vi "setVolumeCount.vi"(8 "error in (no error)":errorcluster, 10 "VolumeCount":u32, 11 "VGS_Project in":refnum<class "VGS_Project.lvclass">) -> (0 "error out":errorcluster, 3 "VGS_Project out":refnum<class "VGS_Project.lvclass">)   [LabVIEW 2022 SP3, in "LV_VGS.lvlib" / "VGS_Project.lvclass"]
uses:
  VGS_Project.lvclass
  VGS_Project.lvclass/VGS_Project.ctl
  C:/Users/Andrey/Desktop/hajo/LV_VGS/vgs_project.dll
  vgs_project.dll
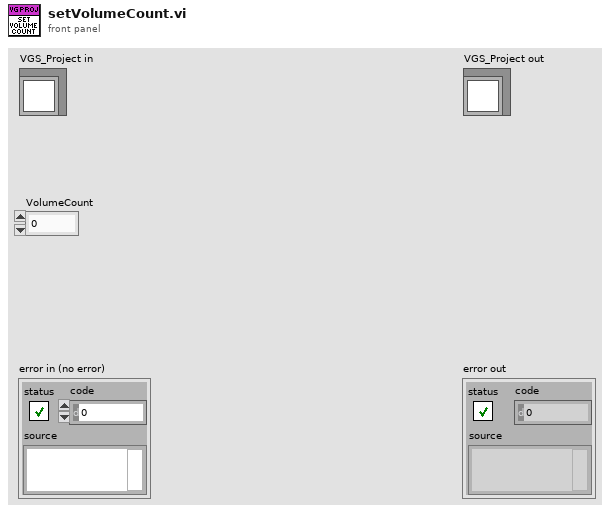
[diagram p1: front panel]
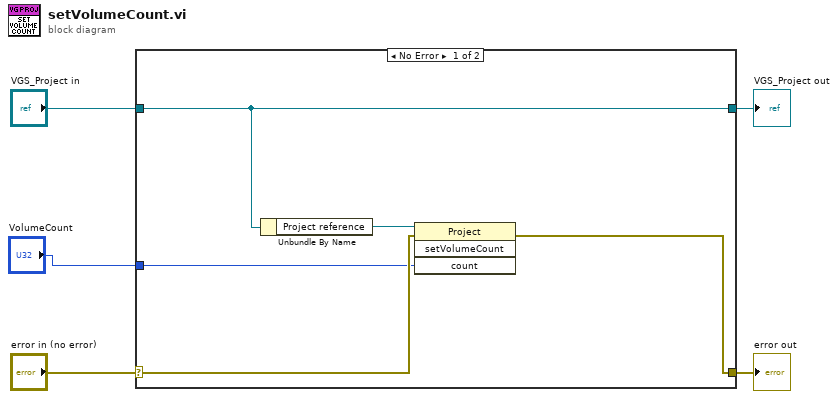
[diagram p0: block diagram]
diagram:
  n1 = case shown="No Error" "error in (no error)" {
    selector: "error in (no error)" -> [w8 w12]
    tunnel: [w7 w12] -> w4
    tunnel: [w10 w11] -> w2
    tunnel: "VGS_Project in" -> [w10 w11]
    tunnel: "VolumeCount" -> [w6 _]
    frame No Error {
      n2 = Unbundle By Name(w10) -> ("Project reference"=w9:refnum<k24>)
      n3 = invoke class="Project" method="setVolumeCount"(reference=w9, error in=w8, "count"=w6) -> (error out=w7:errorcluster)  [unwired: 1 in, 3 out]
    }
    frame Error {
    }
  }
  "error out" <- w4
  "VGS_Project out" <- w2
